vi "get camera register timestamp from harp .bin file.vi"(3 "harp .bin":path, 4 "reference 4":refnum<vi>, 5 "reference 3":refnum<vi>, 6 "reference 2":refnum<vi>, 7 "reference":refnum<vi>) -> (0 "Array":dbl[](array[numeric]), 1 "Abort":bool)   [LabVIEW 2010]
panel:
  out "Array 2":bool[](array[boolean])
  out "x+y":u32
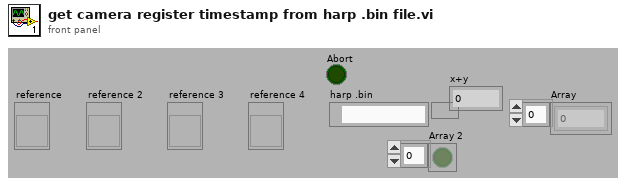
[diagram p1: front panel]
types:
  T1 = enum16{"open", "replace", "create", "open or create", "replace or create", "replace or create with confirmation"}
  T2 = enum16{"CreateBuffer", "WriteBytes", "WriteByte", "AvailableMemory", "OccupiedMemory", "CheckBytes", "ReadBytes"}
  T3 = cluster{"Timestamp(us)":dbl, "Command":u8, "Error":bool, "Register Address":u8, "Port":u8, "Number of Elements":u8, "Type":u8, "I8":i8, "U8":u8, "U16":u16, "I16":i16, "U32":u32, "I32":i32, "U64":u64, "I64":i64, "Float":sgl, "U8[]":u8[], "I8[]":i8[], "U16[]":u16[], "I16[]":i16[], "U32[]":u32[], "I32[]":i32[], "U64[]":u64[], "I64[]":i64[], "Float[]":sgl[]}
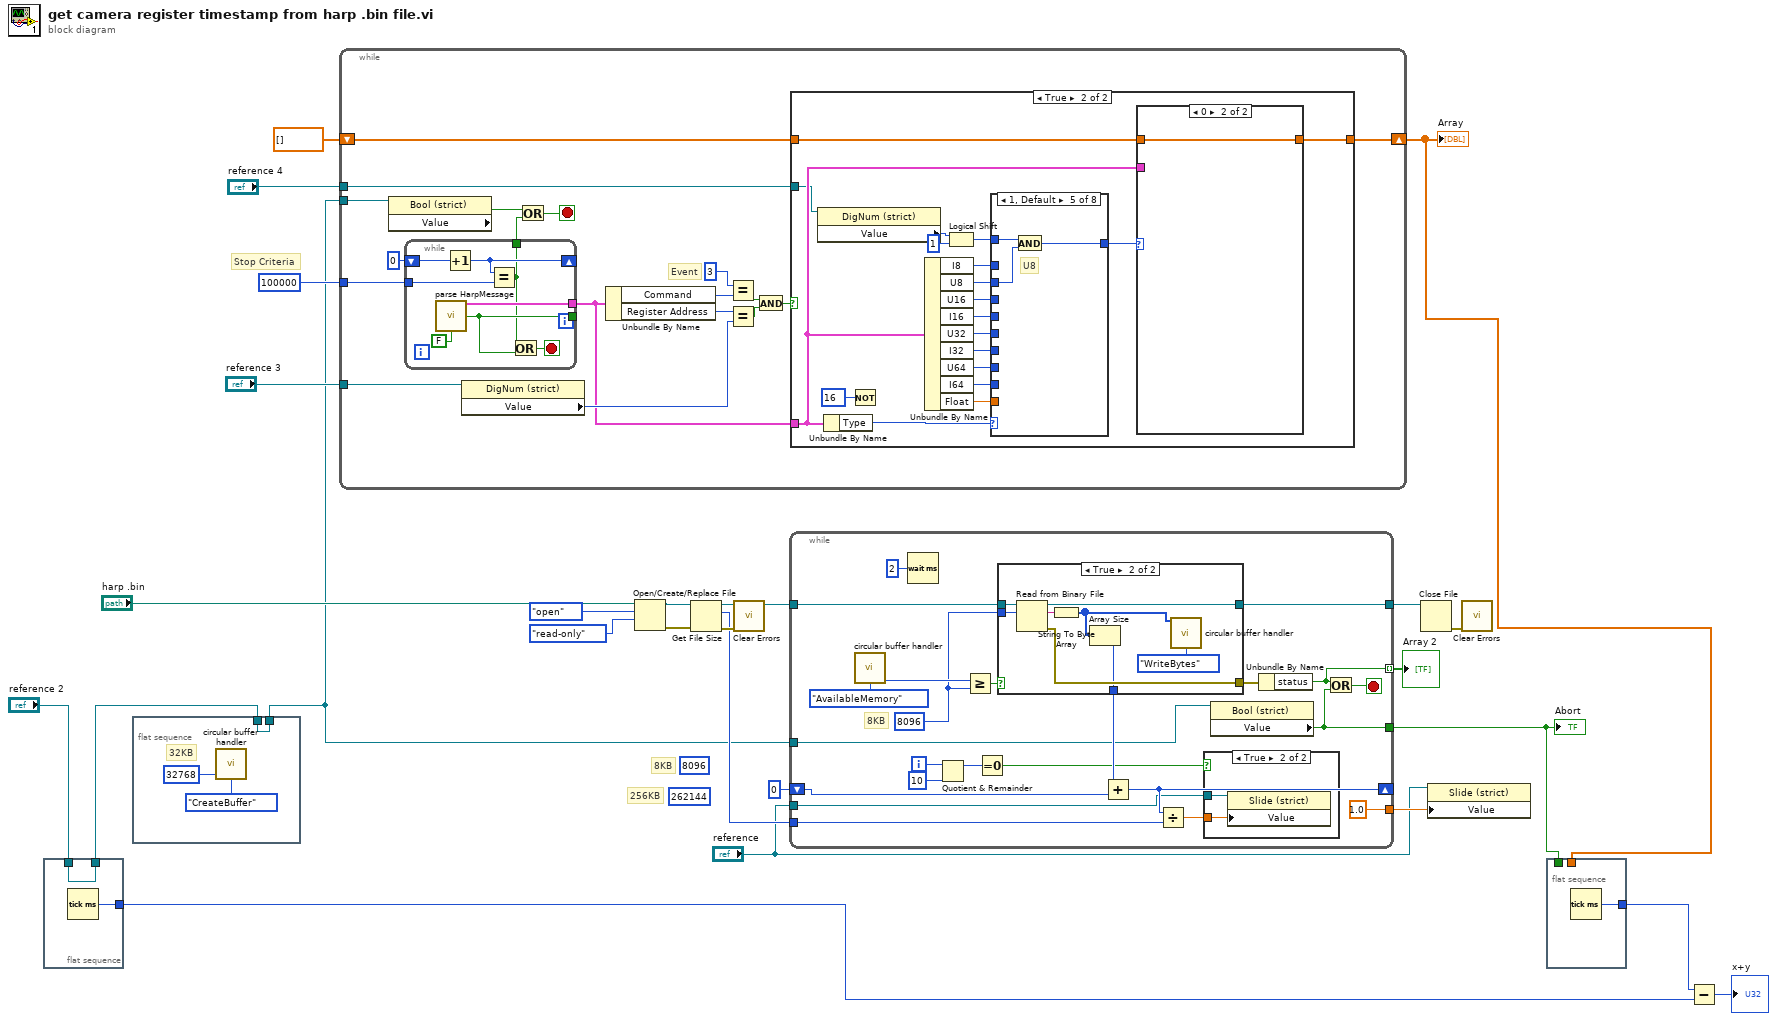
[diagram p0: block diagram]
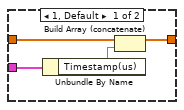
[diagram p3: hidden frame]
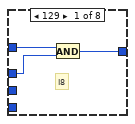
[diagram p4: hidden frame]
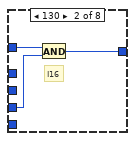
[diagram p5: hidden frame]
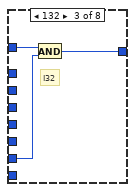
[diagram p6: hidden frame]
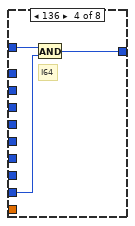
[diagram p7: hidden frame]
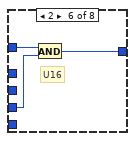
[diagram p8: hidden frame]
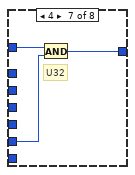
[diagram p9: hidden frame]
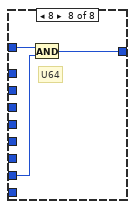
[diagram p10: hidden frame]
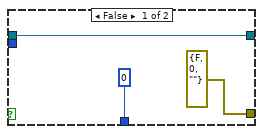
[diagram p12: hidden frame]
diagram:
  (unwired) 262144 ("y")
  (unwired) 8096 ("y")
  # "Stop Criteria"
  # "256KB"
  # "8KB"
  n1 = flat-sequence {
    tunnel: [w28] -> w7
    tunnel: "reference 2" -> [w28]
    tunnel: [w27] -> w5
    frame #0 {
      n2 = Tick Count (ms)() -> (millisecond timer value=w27:u32)
    }
  }
  n3 = flat-sequence {
    tunnel: [w30] -> w9
    tunnel: w7 -> [w30]
    frame #0 {
      # "32KB"
      n4 = call "circular buffer handler.vi"("NumberOfBytes"=32768, "Enum"=T2."CreateBuffer") -> ()  [unwired: 11 in, 3 out]
    }
  }
  n5 = while {
    tunnel: 100000 ("NumberOfBytes") -> [w48]
    shift-right: [w35] -> w3
    shift-left: dbl[] [] ("Array") -> [w36]
    tunnel: w9 -> [w34]
    tunnel: "reference 3" -> [w33]
    tunnel: "reference 4" -> [w32]
    stop <- w46 stop-if-true
    # "Event"
    n6 = property class="Bool (strict)"(reference=w34) -> ("Value"=w45:bool)  [unwired: 1 in, 2 out]
    n7 = while {
      tunnel: [w106] -> w40
      tunnel: [w105] -> _
      shift-right: [w103] -> _
      shift-left: 0 ("NumberOfBytes") -> [w104]
      tunnel: w48 -> [w102]
      tunnel: [w100] -> w47
      stop <- w101 stop-if-true
      n8 = call "parse HarpMessage.vi"("Round value"=FALSE) -> ("HarpDataFrame"=w106:T3, "Packet Found"=w105:bool)  [unwired: 12 in, 1 out]
      n9 = Increment(x=w104) -> (x+1=w103:i32)
      n10 = Equal?(x=w103, y=w102) -> (x = y?=w100:bool)
      n11 = Or(x=w100, y=w105) -> (x .or. y?=w101:bool)
    }
    n12 = property class="DigNum (strict)"(reference=w33) -> ("Value"=w41:i32)  [unwired: 1 in, 2 out]
    n13 = Or(x=w45, y=w47) -> (x .or. y?=w46:bool)
    n14 = Unbundle By Name(w40) -> ("Command"=w44:u8, "Register Address"=w42:u8)
    n15 = Equal?(x=u8 3, y=w44) -> (x = y?=w38:bool)
    n16 = Equal?(x=w42, y=w41) -> (x = y?=w39:bool)
    n17 = And(x=w38, y=w39) -> (x .and. y?=w37:bool)
    n18 = case shown="True" w37 {
      tunnel: w40 -> [_ w56]
      tunnel: w36 -> [w50 w55]
      tunnel: [w50 w54] -> w35
      tunnel: w32 -> [_ w52]
      frame False {
      }
      frame True {
        n19 = property class="DigNum (strict)"(reference=w52) -> ("Value"=w66:i32)  [unwired: 1 in, 2 out]
        n20 = Unbundle By Name(w56) -> ("Type"=w51:u8)
        n21 = Not(x=u8 16) -> ()  [unwired: 1 out]
        n22 = Unbundle By Name(w56) -> ("I8"=w57:i8, "U8"=w58:u8, "U16"=w59:u16, "I16"=w60:i16, "U32"=w61:u32, "I32"=w62:i32, "U64"=w63:u64, "I64"=w64:i64, "Float"=w65:sgl)
        n23 = Logical Shift(y=w66, x=1) -> (x << y=w68:i32)
        n24 = case shown="1, Default" w51 {
          tunnel: w57 -> [w76 _ _ _ _ _ _ _]
          tunnel: w58 -> [_ _ _ _ w88 _ _ _]
          tunnel: w59 -> [_ w79 _ _ _ w92 _ _]
          tunnel: w60 -> [_ _ _ _ _ _ _ _]
          tunnel: w61 -> [_ _ _ _ _ _ w94 _]
          tunnel: w62 -> [_ _ w82 _ _ _ _ _]
          tunnel: w63 -> [_ _ _ _ _ _ _ w97]
          tunnel: w64 -> [_ _ _ w85 _ _ _ _]
          tunnel: w65 -> [_ _ _ _ _ _ _ _]
          tunnel: w68 -> [w77 w80 w83 w86 w89 w91 w95 w98]
          tunnel: [w75 w78 w81 w84 w87 w90 w93 w96] -> w53
          frame 129 {
            # "I8"
            n25 = And(x=w77, y=w76) -> (x .and. y?=w75:i32)
          }
          frame 130 {
            # "I16"
            n26 = And(x=w80, y=w79) -> (x .and. y?=w78:i32)
          }
          frame 132 {
            # "I32"
            n27 = And(x=w83, y=w82) -> (x .and. y?=w81:i32)
          }
          frame 136 {
            # "I64"
            n28 = And(x=w86, y=w85) -> (x .and. y?=w84:i64)
          }
          frame 1, Default {
            # "U8"
            n29 = And(x=w89, y=w88) -> (x .and. y?=w87:i32)
          }
          frame 2 {
            # "U16"
            n30 = And(x=w91, y=w92) -> (x .and. y?=w90:i32)
          }
          frame 4 {
            # "U32"
            n31 = And(x=w95, y=w94) -> (x .and. y?=w93:u32)
          }
          frame 8 {
            # "U64"
            n32 = And(x=w98, y=w97) -> (x .and. y?=w96:u64)
          }
        }
        n33 = case shown="0" w53 {
          tunnel: w56 -> [w73 _]
          tunnel: w55 -> [w72 w74]
          tunnel: [w70 w74] -> w54
          frame 1, Default {
            n34 = Unbundle By Name(w73) -> ("Timestamp(us)"=w71:dbl)
            n35 = Build Array (concatenate)(w72, w71) -> (w70:dbl[])
          }
          frame 0 {
          }
        }
      }
    }
  }
  "Array" <- w3
  n36 = Open/Create/Replace File(file path (use dialog)="harp .bin", operation (0:open)=T1."open", access (0:read/write)=enum16{"read/write", "read-only", "write-only"}."read-only") -> (refnum out=w21:refnum<file>, error out=w10:errorcluster)  [unwired: 3 in, 1 out]
  n37 = Get File Size(file=w21, error in=w10) -> (refnum out=w17:refnum<file>, size (in bytes)=w14:i64, 0:w16:errorcluster)
  n38 = call <vilib>:"Clear Errors.vi"("error in (no error)"=w16) -> ()  [unwired: 6 in, 1 out]
  n39 = while {
    tunnel: w17 -> [w128]
    tunnel: [w127] -> w18
    shift-right: [w124] -> _
    shift-left: 0 -> [w125]
    tunnel: w14 -> [w123]
    tunnel: [1.0 ("Creating CSV")] -> w25
    tunnel: "reference" -> [w111]
    tunnel: w9 -> [w110]
    tunnel: [w109] -> w2
    tunnel: [w107] -> w1 mode=indexing
    i -> [w119]
    stop <- w112 stop-if-true
    w108 = 8096 ("y")
    # "8KB"
    n40 = call "circular buffer handler.vi"("Enum"=T2."AvailableMemory") -> ("Output"=w121:i32)  [unwired: 12 in, 2 out]
    n41 = Wait (ms)(milliseconds to wait=u32 2) -> ()  [unwired: 1 out]
    n42 = Quotient & Remainder(x=w119, y=10) -> (x-y*floor(x/y)=w117:i32)  [unwired: 1 out]
    n43 = Greater Or Equal?(x=w121, y=w108) -> (x >= y?=w115:bool)
    n44 = Equal To 0?(x=w117) -> (x = 0?=w114:bool)
    n45 = case shown="True" w115 {
      tunnel: w128 -> [w134 w142]
      tunnel: w108 -> [_ w141]
      tunnel: [errorcluster {"status"=FALSE, "code"=0, "source"=""} ("error out") w138] -> w113
      tunnel: [w134 w137] -> w127
      tunnel: [0 w135] -> w126
      frame False {
      }
      frame True {
        n46 = Read from Binary File(10:w141, 11:w142) -> (0:w138:errorcluster, 2:w140:string, 3:w137:refnum<file>)  [unwired: 4 in, 1 out]
        n47 = String To Byte Array(string=w140) -> (unsigned byte array=w136:u8[])
        n48 = Array Size(array=w136) -> (size(s)=w135:i32)
        n49 = call "circular buffer handler.vi"("StreamToWrite"=w136, "Enum"=T2."WriteBytes") -> ()  [unwired: 11 in, 3 out]
      }
    }
    n50 = Add(x=w126, y=w125) -> (x+y=w124:i32)
    n51 = Divide(x=w124, y=w123) -> (x/y=w122:dbl)
    n52 = case shown="True" w114 {
      tunnel: w122 -> [_ w131]
      tunnel: w111 -> [_ w130]
      frame False {
      }
      frame True {
        n53 = property class="Slide (strict)"(reference=w130, "Value"=w131) -> ()  [unwired: 1 in, 2 out]
      }
    }
    n54 = property class="Bool (strict)"(reference=w110) -> ("Value"=w109:bool)  [unwired: 1 in, 2 out]
    n55 = Unbundle By Name(w113) -> ("status"=w107:bool)
    n56 = Or(x=w107, y=w109) -> (x .or. y?=w112:bool)
  }
  "Abort" <- w2
  "Array 2" <- w1
  n57 = Close File(refnum=w18) -> (error out=w26:errorcluster)  [unwired: 1 in, 1 out]
  n58 = property class="Slide (strict)"(reference="reference", "Value"=w25) -> ()  [unwired: 1 in, 2 out]
  n59 = call <vilib>:"Clear Errors.vi"("error in (no error)"=w26) -> ()  [unwired: 6 in, 1 out]
  n60 = flat-sequence {
    tunnel: w3 -> [_]
    tunnel: [w143] -> w6
    tunnel: w2 -> [_]
    frame #0 {
      n61 = Tick Count (ms)() -> (millisecond timer value=w143:u32)
    }
  }
  n62 = Subtract(x=w6, y=w5) -> (x-y=→"x+y":u32)
